vi "Asynchronous Call.vi"() -> ()   [LabVIEW 2020, in "Multi Process.lvlib"]
uses:
  Multi Process.lvlib
  f501469e-a2b6-4afe-80ea-40ced5d70a01.vi
  Msg Handler.vi
panel:
  in  "stop":bool
  in  "Exe":bool
  in  "Init":bool
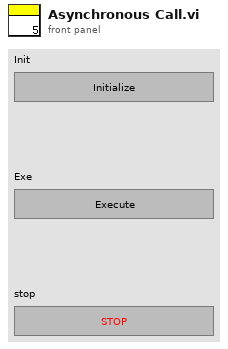
[diagram p1: front panel]
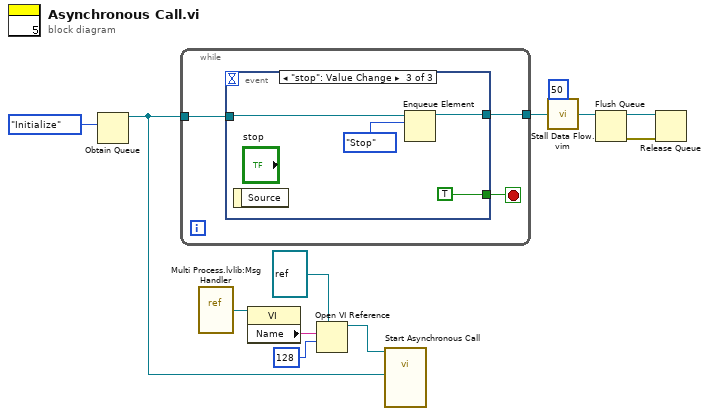
[diagram p0: block diagram]
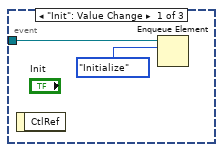
[diagram p2: hidden frame]
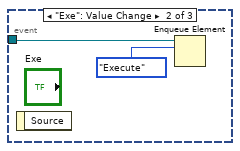
[diagram p3: hidden frame]
diagram:
  n1 = Obtain Queue(element data type=enum16{"Stop", "Execute", "Initialize"}."Initialize") -> (queue out=w5:refnum<queue>)  [unwired: 4 in, 2 out]
  n2 = while {
    tunnel: w5 -> [w15]
    tunnel: [w13] -> w3
    stop <- w14 stop-if-true
    n3 = event shown="[2] \"stop\": Value Change" {
      selector: _ -> [_ _ _]
      dyn-events: _ -> [_ _ _]
      timeout: _ -> [_ _ _]
      tunnel: w15 -> [w17 w18 w22]
      tunnel: [_ _ TRUE] -> w14
      tunnel: [_ _ w20] -> w13
      event "Init": Value Change {
        n4 = event-data() -> ()  [unwired: 1 in, 1 out]
        n5 = Enqueue Element(queue=w17, element=enum16{"Stop", "Execute", "Initialize"}."Initialize") -> ()  [unwired: 2 in, 3 out]
      }
      event "Exe": Value Change {
        n6 = event-data() -> ()  [unwired: 1 in, 1 out]
        n7 = Enqueue Element(queue=w18, element=enum16{"Stop", "Execute", "Initialize"}."Execute") -> ()  [unwired: 2 in, 3 out]
      }
      event "stop": Value Change {
        n8 = event-data() -> ()  [unwired: 1 in, 1 out]
        n9 = Enqueue Element(queue=w22, element=enum16{"Stop", "Execute", "Initialize"}."Stop") -> (queue out=w20:refnum<queue>)  [unwired: 2 in, 2 out]
      }
    }
  }
  n10 = vi-ref "Multi Process.lvlib:Msg Handler.vi"() -> (w7:refnum<vi>)
  n11 = property class="VI"(reference=w7) -> ("Name"=w6:string)  [unwired: 1 in, 2 out]
  n12 = Open VI Reference(type specifier VI Refnum (for type only)=refnum<vi> refnum, vi path=w6, options=128) -> (vi reference=w9:refnum<vi>)  [unwired: 3 in, 1 out]
  n13 = call-by-ref "Start Asynchronous Call"(reference=w9, "queue"=w5) -> ()  [unwired: 11 in, 3 out]
  n14 = call "Stall Data Flow.vim"("value in"=w3, "milliseconds to wait"=u32 50) -> ("value out"=w2:refnum<queue>)  [unwired: 1 out]
  n15 = Flush Queue(queue=w2) -> (queue out=w10:refnum<queue>, error out=w11:errorcluster)  [unwired: 1 in, 1 out]
  n16 = Release Queue(queue=w10, error in (no error)=w11) -> ()  [unwired: 1 in, 3 out]
